vi "Set Object Pointer.vi"(10 "Object Pointer":i64, 11 "TreeNodeArray in":refnum<class "TreeNodeArray.lvclass">) -> (3 "TreeNodeArray out":refnum<class "TreeNodeArray.lvclass">)   [LabVIEW 2012, in "MDSplus.lvlib" / "TreeNodeArray.lvclass"]
uses:
  <vilib>/MDSplus/Classes/TreeNodeArray_Class/TreeNodeArray.lvclass
  <vilib>/MDSplus/Classes/TreeNodeArray_Class/TreeNodeArray.lvclass/TreeNodeArray.ctl
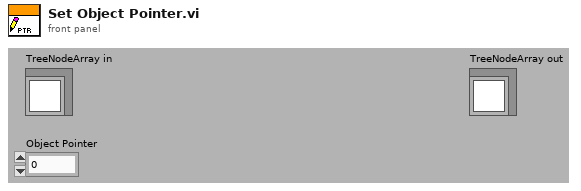
[diagram p1: front panel]
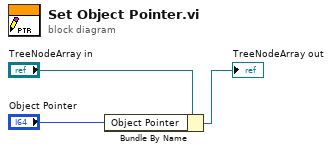
[diagram p0: block diagram]
diagram:
  n1 = Bundle By Name(cluster="TreeNodeArray in", "Object Pointer"="Object Pointer") -> (→"TreeNodeArray out":refnum<class "TreeNodeArray.lvclass">)
